vi "Gamma1.vi"(10 "Value":u32) -> (2 "Gamma 1":u32)   [LabVIEW 2015, in "Crypto.lvlib" / "SHA-256.lvclass"]
uses:
  SHA-256.lvclass
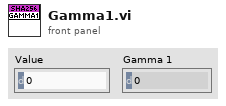
[diagram p1: front panel]
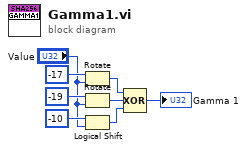
[diagram p0: block diagram]
diagram:
  n1 = Rotate(1:"Value", 2:i16 -17 ("y")) -> (0:w2:u32)
  n2 = Rotate(1:"Value", 2:i16 -19 ("y")) -> (0:w4:u32)
  n3 = Logical Shift(y=i16 -10, x="Value") -> (x << y=w3:u32)
  n4 = Compound Arithmetic op=XOR(w2, w4, w3) -> (→"Gamma 1":u32)
